vi "CV Power Law Fit.vi"(8 "Error In":errorcluster, 9 "Plot":T1, 10 "ICCD Parameter Set":T4, 11 "ICCD Parameter Array":string[][](array[string])) -> (0 "Error Out":errorcluster, 1 "Power Law Fit Results":T2, 3 "Plot Fit":T1)   [LabVIEW 2021, in "AlliGator Camera Noise Influence on Lifetime.lvlib"]
uses:
  AlliGator Camera Noise Influence on Lifetime.lvlib
  ICCD Parameter Set.ctl
  Graphs/XY Graph/XY Graph Plot Data.ctl
  Decay Fit Parameter Map/AlliGator Power Law Fit Results.ctl
  Power Law Parameters.ctl
  <userlib>/_OpenG.lib/array/array.llb/Filter 1D Array with Scalar (DBL)__ogtk.vi
  <userlib>/_OpenG.lib/array/array.llb/Delete Elements from 1D Array (DBL)__ogtk.vi
  <vilib>/gmath/NI_Gmath.lvlib
  <vilib>/Analysis/NI_AALPro.lvlib
  <userlib>/_OpenG.lib/array/array.llb/openg_array.lvlib
  Graphs/XY Graph/XY Graph Add-Ons.lvlib
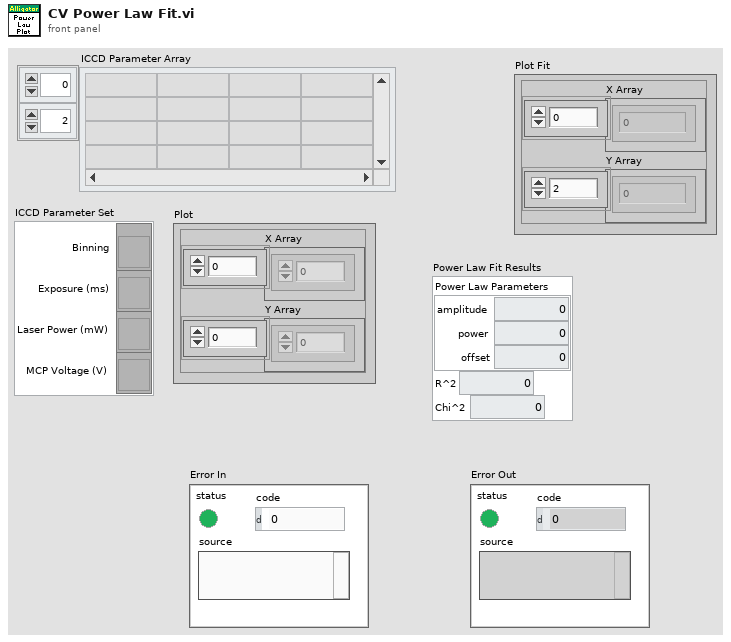
[diagram p1: front panel]
types:
  T1 = typedef "XY Graph Add-Ons.lvlib/XY Graph Plot Data.ctl" = cluster{"X Array":dbl[], "Y Array":dbl[]}
  T2 = typedef "AlliGator Camera Noise Influence on Lifetime.lvlib/AlliGator Power Law Fit Results.ctl" = cluster{"Power Law Parameters":T3, "R^2":dbl, "Chi^2":dbl}
  T3 = typedef "AlliGator Camera Noise Influence on Lifetime.lvlib/Power Law Parameters.ctl" = cluster{"amplitude":dbl, "power":dbl, "offset":dbl}
  T4 = typedef "AlliGator Camera Noise Influence on Lifetime.lvlib/ICCD Parameter Set.ctl" = cluster{"Binning":refnum<vi>, "Exposure (ms)":refnum<vi>, "Laser Power (mW)":refnum<vi>, "MCP Voltage (V)":refnum<vi>}
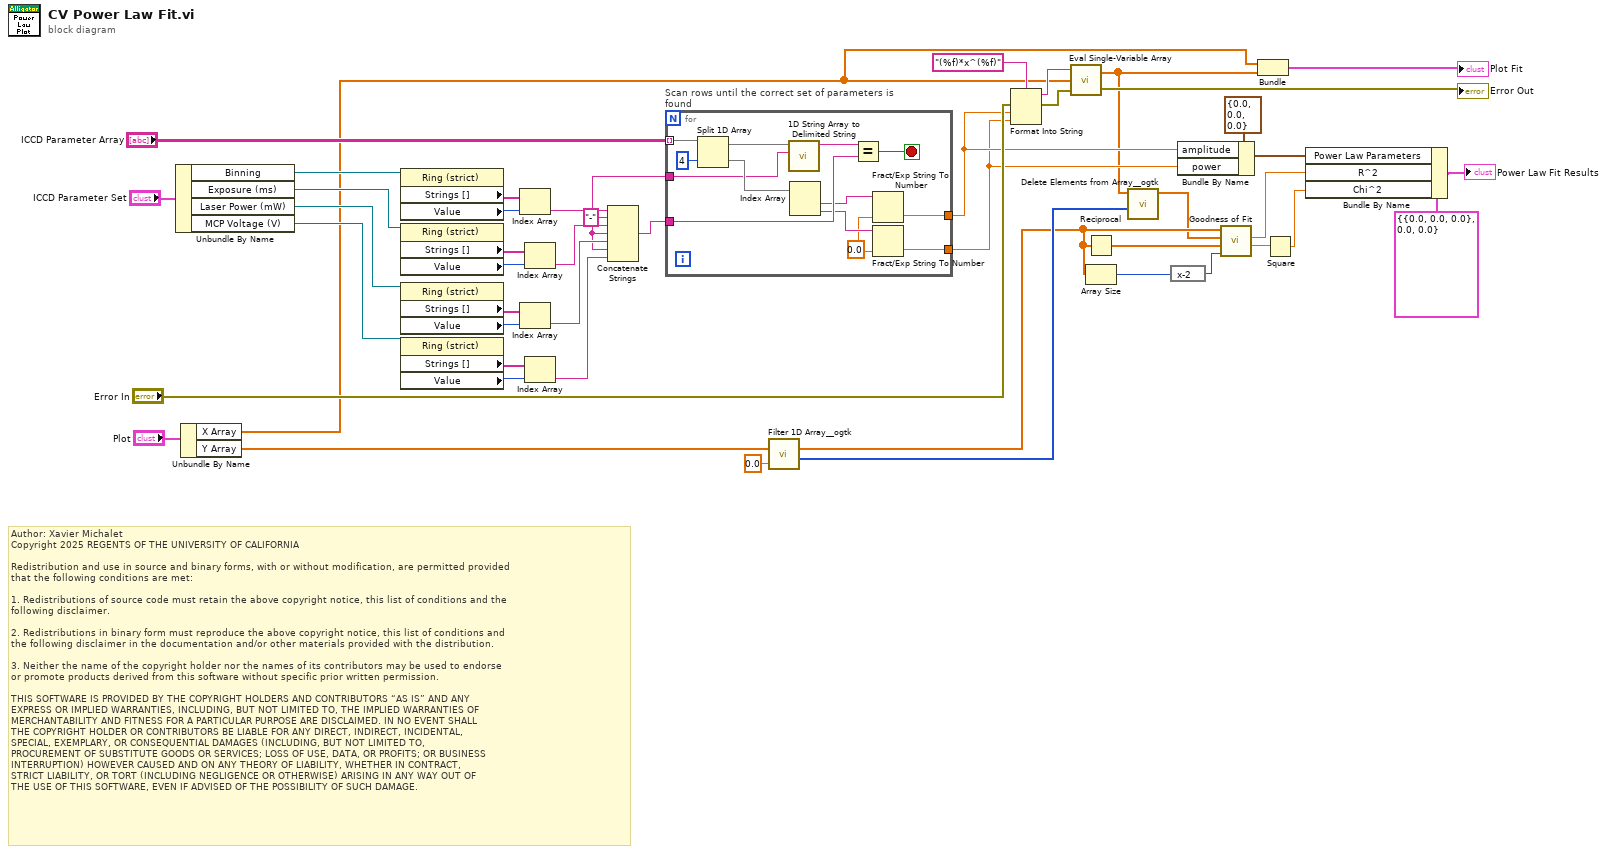
[diagram p0: block diagram]
diagram:
  w20 = "-" ("string")
  # "Author: Xavier Michalet\nCopyright 2025 REGENTS OF THE UNIVERSITY OF CALIFORNIA\n\nRedistribution and use in source and binary forms, with or without modification, are permitted provided\nthat the following conditions are met:\n\n1. Redistributions of source code must retain the above copyright notice, this list of conditions and the\nfollowing disclaimer.\n\n2. Redistributions in binary form must reproduce the above copyright notice, this list of conditions and\nthe following disclaimer in the documentation and/or other materials provided with the distribution.\n\n3. Neither the name of the copyright holder nor the names of its contributors may be used to endorse \nor promote products derived from this software without specific prior written permission.\n\nTHIS SOFTWARE IS PROVIDED BY THE COPYRIGHT HOLDERS AND CONTRIBUTORS “AS IS” AND ANY \nEXPRESS OR IMPLIED WARRANTIES, INCLUDING, BUT NOT LIMITED TO, THE IMPLIED WARRANTIES OF\nMERCHANTABILITY AND FITNESS FOR A PARTICULAR PURPOSE ARE DISCLAIMED. IN NO EVENT SHALL\nTHE COPYRIGHT HOLDER OR CONTRIBUTORS BE LIABLE FOR ANY DIRECT, INDIRECT, INCIDENTAL, \nSPECIAL, EXEMPLARY, OR CONSEQUENTIAL DAMAGES (INCLUDING, BUT NOT LIMITED TO, \nPROCUREMENT OF SUBSTITUTE GOODS OR SERVICES; LOSS OF USE, DATA, OR PROFITS; OR BUSINESS\nINTERRUPTION) HOWEVER CAUSED AND ON ANY THEORY OF LIABILITY, WHETHER IN CONTRACT, \nSTRICT LIABILITY, OR TORT (INCLUDING NEGLIGENCE OR OTHERWISE) ARISING IN ANY WAY OUT OF\nTHE USE OF THIS SOFTWARE, EVEN IF ADVISED OF THE POSSIBILITY OF SUCH DAMAGE."
  n1 = Unbundle By Name("ICCD Parameter Set") -> ("Binning"=w44:refnum<vi>, "Exposure (ms)"=w39:refnum<vi>, "Laser Power (mW)"=w34:refnum<vi>, "MCP Voltage (V)"=w33:refnum<vi>)
  n2 = Unbundle By Name("Plot") -> ("X Array"=w1:dbl[], "Y Array"=w4:dbl[])
  n3 = property class="Ring (strict)"(reference=w44) -> ("Strings []"=w43:string[], "Value"=w42:i32)  [unwired: 1 in, 2 out]
  n4 = property class="Ring (strict)"(reference=w39) -> ("Strings []"=w41:string[], "Value"=w40:i32)  [unwired: 1 in, 2 out]
  n5 = property class="Ring (strict)"(reference=w34) -> ("Strings []"=w35:string[], "Value"=w36:i32)  [unwired: 1 in, 2 out]
  n6 = property class="Ring (strict)"(reference=w33) -> ("Strings []"=w37:string[], "Value"=w38:i32)  [unwired: 1 in, 2 out]
  n7 = Index Array(array=w43, index=w42) -> (element=w32:string)
  n8 = Index Array(array=w35, index=w36) -> (element=w30:string)
  n9 = Index Array(array=w41, index=w40) -> (element=w31:string)
  n10 = Index Array(array=w37, index=w38) -> (element=w29:string)
  n11 = Concatenate Strings(w32, w20, w31, w20, w30, w20, w29) -> (w27:string)
  n12 = for "Scan rows until the correct set of parameters is found" {
    tunnel: "ICCD Parameter Array" -> [w58] mode=indexing
    tunnel: w27 -> [w54]
    tunnel: [w48] -> w19
    tunnel: [w47] -> w18
    tunnel: w20 -> [w46]
    stop <- w53 stop-if-true
    w49 = 0.0 ("default (0 I32)")
    n13 = Split 1D Array(array=w58, index=4) -> (first subarray=w56:string[], second subarray=w52:string[])
    n14 = call <vilib>:"1D String Array to Delimited String.vi"("delimiter"=w46, "string array"=w56) -> ("delimited string"=w55:string)  [unwired: 9 in]
    n15 = Index Array(array=w52) -> (element #1=w51:string, element #2=w50:string)  [unwired: 2 in]
    n16 = Equal?(x=w55, y=w54) -> (x = y?=w53:bool)
    n17 = Fract/Exp String To Number(string=w51, default (0 dbl)=w49) -> (number=w48:dbl)  [unwired: 2 in, 1 out]
    n18 = Fract/Exp String To Number(string=w50, default (0 dbl)=w49) -> (number=w47:dbl)  [unwired: 2 in, 1 out]
  }
  n19 = call-poly <userlib>:"Filter 1D Array__ogtk.vi"("items to filter"=0.0, "array"=w4) -> ("filtered item indices"=w5:i32[])  [unwired: 4 in, 1 out]
  n20 = Format Into String(format string="(%f)*x^(%f)", error in="Error In", w19, w18) -> (resulting string=w25:string, error out=w26:errorcluster)  [unwired: 1 in]
  n21 = call <vilib>:"Eval Single-Variable Array.vi"("error in (no error)"=w26, "X Values"=w1, "formula"=w25) -> ("error out"=→"Error Out":errorcluster, "Y Values"=w3:dbl[])
  n22 = Reciprocal(x=w4) -> (1/x=w12:dbl[])
  n23 = Array Size(array=w4) -> (size(s)=w11:i32)
  n24 = call-poly <userlib>:"Delete Elements from Array__ogtk.vi"("indices"=w5, "array"=w3) -> ("array w/ subset deleted"=w2:dbl[])  [unwired: 8 in, 1 out]
  n25 = expression code="x-2"(w11) -> (w10:i32)
  n26 = Bundle By Name(cluster=T3 {"amplitude"=0.0, "power"=0.0, "offset"=0.0} ("Power Law Parameters"), "amplitude"=w19, "power"=w18) -> (w16:T3)
  n27 = call <vilib>:"Goodness of Fit.vi"("degree of freedom"=w10, "Weight"=w12, "Best Fit"=w2, "Y"=w4) -> ("RMSE"=w8:dbl, "R-square"=w9:dbl)  [unwired: 4 in, 2 out]
  n28 = Bundle("X Array"=w1, "Y Values"=w3) -> (→"Plot Fit":cluster{"X Array":dbl[], "Y Values":dbl[]})  [unwired: 1 in]
  n29 = Square(x=w8) -> (x^2=w7:dbl)
  n30 = Bundle By Name(cluster=T2 {"Power Law Parameters"={"amplitude"=0.0, "power"=0.0, "offset"=0.0}, "R^2"=0.0, "Chi^2"=0.0} ("Power Law Fit Results"), "Power Law Parameters"=w16, "R^2"=w9, "Chi^2"=w7) -> (→"Power Law Fit Results":T2)
